vi "ShutDown.vi"(8 "error in":errorcluster, 11 "Laser in":refnum<class "Laser.lvclass">) -> (0 "error out":errorcluster, 3 "Laser out":refnum<class "Laser.lvclass">)   [LabVIEW 2018, in "Laser.lvlib" / "Laser.lvclass"]
uses:
  Laser.lvclass
  Custom Controls/Command List.ctl
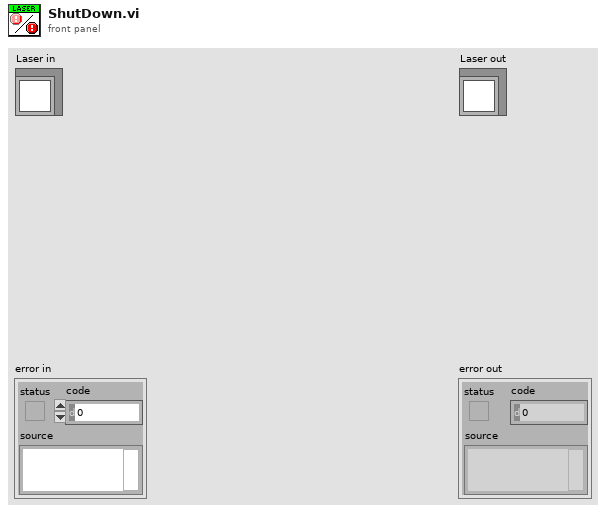
[diagram p1: front panel]
types:
  T1 = typedef "Laser.lvlib/Laser.lvclass/Command List.ctl" = enum16{"None", "Config?", "Volt?", "ThCase?", "STS?", "Mon?", "Help?", "HB", "Verbose", "Spnt", "Ext", "PRF", "Start", "Stop", "PRF?", "State?", "Status?", "Stat?", "Read HB", "Logon", "Poutmax", "saveconfig", "Reset", "Poutmax?", "PoutCommandMax", "PoutCommandMax?", "FreqMin", "FreqMin?"}
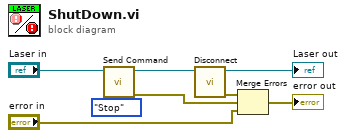
[diagram p0: block diagram]
diagram:
  n1 = call-dynamic "Send Command.vi"("Command in"=Command_List."Stop" ("Command"), "Laser in"="Laser in") -> ("error out"=w2:errorcluster, "Laser out"=w5:refnum<class "Laser.lvclass">)  [unwired: 7 in, 1 out]
  n2 = call-dynamic "Disconnect.vi"("Laser in"=w5) -> ("error out"=w4:errorcluster, "Laser out"=→"Laser out":refnum<class "Laser.lvclass">)  [unwired: 9 in]
  n3 = Merge Errors(w4, w2, "error in") -> (→"error out":errorcluster)
